vi "AFT Get Coefficients.vi"   [LabVIEW 2017, in "NI_AdaptiveFilter.lvlib"]
doc: "Retrieves the filter coefficients from an adaptive filter that you create with the least mean squares (LMS) or recursive least squares (RLS) algorithms. You must manually select the polymorphic instance you want to use."
uses:
  <vilib>/addons/Adaptive Filters/NI_AdaptiveFilter.lvlib
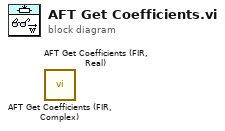
[diagram p0: block diagram]
diagram:
  n1 = call <vilib>:"AFT Get Coefficients (FIR, Complex).vi"() -> ()  [unwired: 9 in, 3 out]
  n2 = call <vilib>:"AFT Get Coefficients (FIR, Real).vi"() -> ()  [unwired: 9 in, 3 out]
